vi "Dbl Array_Linearize NAN values.vi"(10 "Digital":bool, 11 "Dbl Array":dbl[](array[numeric])) -> (2 "Success Out":bool=TRUE, 3 "Dbl Array Out":dbl[](array[numeric]))   [LabVIEW 2024]
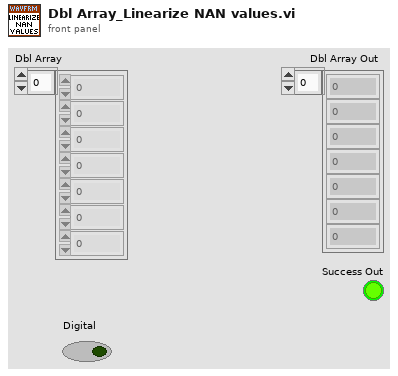
[diagram p1: front panel]
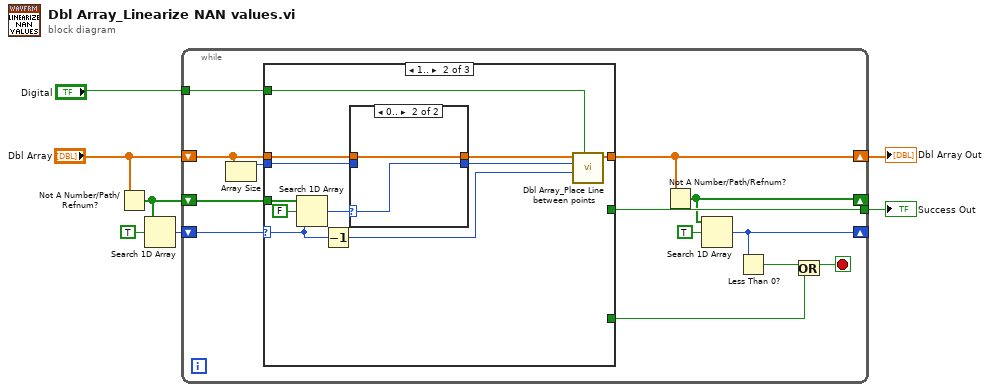
[diagram p0: block diagram]
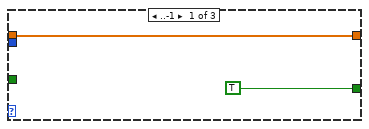
[diagram p2: hidden frame]
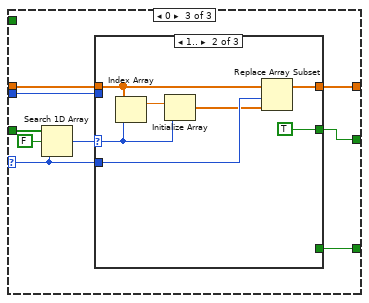
[diagram p4: hidden frame]
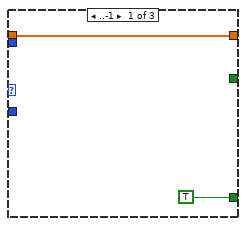
[diagram p5: hidden frame]
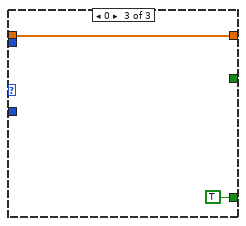
[diagram p6: hidden frame]
diagram:
  n1 = Not A Number/Path/Refnum?(number/path/refnum="Dbl Array") -> (NaN/Path/Refnum?=w3:bool[])
  n2 = Search 1D Array(1D array=w3, element=TRUE) -> (index of element=w2:i32)  [unwired: 1 in]
  n3 = while {
    shift-right: [w14] -> w7
    shift-left: "Dbl Array" -> [w19]
    tunnel: [w20] -> w6
    shift-right: [w12] -> _
    shift-left: w3 -> [w17]
    shift-right: [w11] -> _
    shift-left: w2 -> [w16]
    tunnel: "Digital" -> [w10]
    stop <- w9 stop-if-true
    n4 = Array Size(array=w19) -> (size(s)=w18:i32)
    n5 = case shown="1.." w16 {
      selector: w16 -> [_ w27 w40]
      tunnel: w19 -> [w22 w30 w43]
      tunnel: w17 -> [_ w33 w46]
      tunnel: [TRUE _ w39] -> w20
      tunnel: [w22 w28 w41] -> w14
      tunnel: w18 -> [_ w25 w42]
      tunnel: w10 -> [_ w23 _]
      tunnel: [_ _ w38] -> w8
      frame ..-1 {
      }
      frame 1.. {
        n6 = Search 1D Array(1D array=w33, element=FALSE, start index (0)=w27) -> (index of element=w31:i32)
        n7 = Decrement(x=w27) -> (x-1=w24:i32)
        n8 = case shown="0.." w31 {
          selector: w31 -> [_ w36]
          tunnel: w30 -> [w35 w37]
          tunnel: [w35 w37] -> w29
          tunnel: [w34 w36] -> w26
          tunnel: w25 -> [w34 _]
          frame ..-1 {
          }
          frame 0.. {
          }
        }
        n9 = call "Dbl Array_Place Line between points.vi"("Digital"=w23, "Second Index"=w24, "First Index"=w26, "Dbl Array"=w29) -> ("Dbl Array Out"=w28:dbl[])  [unwired: 7 in]
      }
      frame 0 {
        n10 = Search 1D Array(1D array=w46, element=FALSE, start index (0)=w40) -> (index of element=w44:i32)
        n11 = case shown="1.." w44 {
          selector: w44 -> [_ w51 _]
          tunnel: w43 -> [w48 w55 w57]
          tunnel: [w48 w53 w57] -> w41
          tunnel: w42 -> [_ _ _]
          tunnel: w40 -> [_ w52 _]
          tunnel: [_ TRUE _] -> w39
          tunnel: [TRUE _ TRUE] -> w38
          frame ..-1 {
          }
          frame 1.. {
            n12 = Index Array(array=w55, index=w51) -> (element=w54:dbl)
            n13 = Initialize Array(w54, w51) -> (w50:dbl[])
            n14 = Replace Array Subset(array=w55, new element=w50, index=w52) -> (w53:dbl[])
          }
          frame 0 {
          }
        }
      }
    }
    n15 = Not A Number/Path/Refnum?(number/path/refnum=w14) -> (NaN/Path/Refnum?=w12:bool[])
    n16 = Search 1D Array(1D array=w12, element=TRUE) -> (index of element=w11:i32)  [unwired: 1 in]
    n17 = Less Than 0?(x=w11) -> (x < 0?=w15:bool)
    n18 = Or(x=w15, y=w8) -> (x .or. y?=w9:bool)
  }
  "Dbl Array Out" <- w7
  "Success Out" <- w6
